vi "RP block write.vi"(8 "Error In":errorcluster, 10 "Data":i16[](array[numeric]), 11 "connection ID":refnum<k5>) -> (0 "Error Out":errorcluster, 3 "connection ID out":refnum<k5>)   [LabVIEW 2016]
uses:
  RP Command.ctl
  RP Write Command TCP.vi
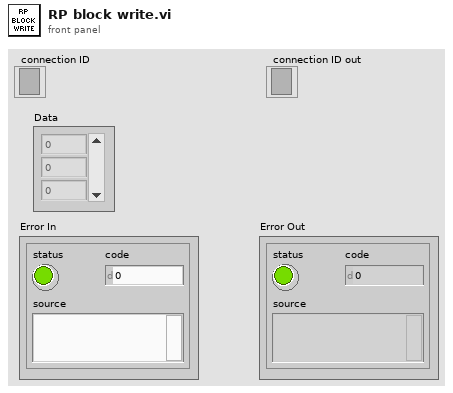
[diagram p1: front panel]
types:
  T1 = typedef "RP Command.ctl" = enum16{"Reset", "Read IDN", "Stop server", "Get status", "Get temperature", "Connect client", "Arm", "Software trigger", "Get whole buffer", "Get chunk", "System call", "Get config", "Set config", "Recieve data", "Play pattern", "Transmit data"}
  T2 = enum16{"big-endian, network order", "native, host order", "little-endian"}
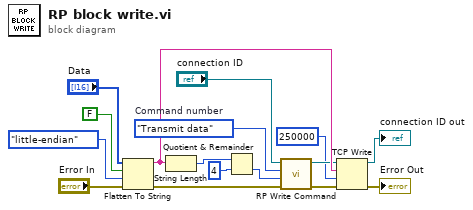
[diagram p0: block diagram]
diagram:
  w5 = RP_Command."Transmit data"  # Command number
  n1 = Flatten To String(anything="Data", prepend array or string size? (T)=FALSE, byte order (0:big-endian, network order)=T2."little-endian", error in (no error)="Error In") -> (data string=w12:string, error out=w7:errorcluster)  [unwired: 1 out]
  n2 = String Length(string=w12) -> (length=w2:i32)
  n3 = Quotient & Remainder(x=w2, y=4) -> (floor(x/y)=w3:i32)  [unwired: 1 out]
  n4 = call-poly "RP Write Command.vi"("Error In"=w7, "Command payload"=w3, "Command number"=w5, "connection ID"="connection ID") -> ("Error Out"=w6:errorcluster, "connection ID out"=w11:refnum<k5>)  [unwired: 5 in, 1 out]
  n5 = TCP Write(connection ID=w11, data in=w12, error in (no error)=w6, 9:250000 ("timeout ms (25000)")) -> (connection ID out=→"connection ID out":refnum<k5>, error out=→"Error Out":errorcluster)  [unwired: 1 out]
